vi "Process_BeamProfileGateSweep.vi"(5 "Gate Start":dbl, 7 "Gate Width":dbl, 9 "Image":dbl[][][](array[numeric])) -> (6 "Gate Delay Array":dbl[](array[numeric]), 8 "Avg Power each frame":dbl[](array[numeric]), 10 "Gate Delay of peak intensity":dbl)   [LabVIEW 2018]
uses:
  <vilib>/Analysis/baseanly.llb/Mean (DBL).vi
  <vilib>/Analysis/NI_AALBase.lvlib
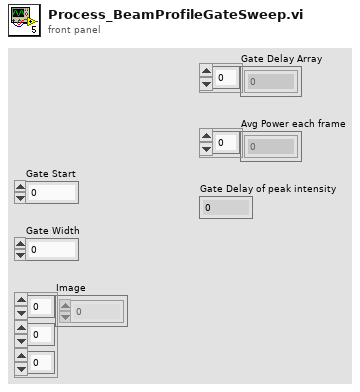
[diagram p1: front panel]
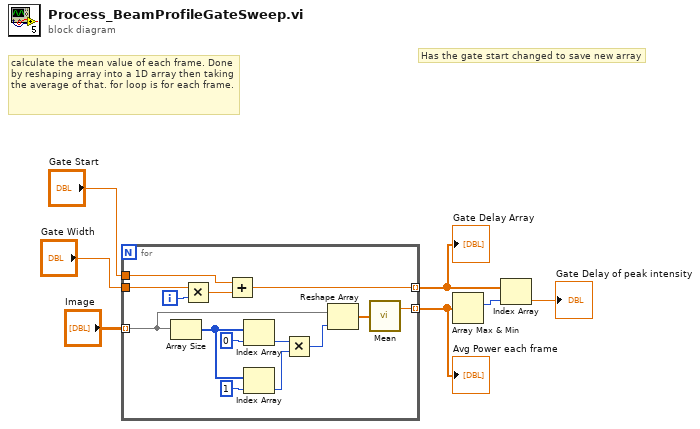
[diagram p0: block diagram]
diagram:
  # "Has the gate start changed to save new array"
  # "calculate the mean value of each frame. Done by reshaping array into a 1D array then taking the average of that. for loop is for each frame."
  n1 = for {
    tunnel: "Image" -> [w14] mode=indexing
    tunnel: [w21] -> w4 mode=indexing
    tunnel: "Gate Start" -> [w17]
    tunnel: "Gate Width" -> [w19]
    tunnel: [w16] -> w5 mode=indexing
    i -> [w20]
    n2 = Array Size(array=w14) -> (size(s)=w13:i32[])
    n3 = Multiply(x=w19, y=w20) -> (x*y=w18:dbl)
    n4 = Add(x=w17, y=w18) -> (x+y=w16:dbl)
    n5 = Index Array(array=w13, index=0) -> (element=w10:i32)
    n6 = Index Array(array=w13, index=1) -> (element=w9:i32)
    n7 = Multiply(x=w10, y=w9) -> (x*y=w8:i32)
    n8 = Reshape Array(w14, w8) -> (w15:dbl[])
    n9 = call-poly <vilib>:"Mean.vi"("X"=w15) -> ("mean"=w21:dbl)  [unwired: 1 out]
  }
  "Gate Delay Array" <- w5
  "Avg Power each frame" <- w4
  n10 = Array Max & Min(array=w4) -> (max index (indices)=w2:i32)  [unwired: 3 out]
  n11 = Index Array(array=w5, index=w2) -> (element=→"Gate Delay of peak intensity":dbl)
